vi "Stop.vi"(8 "error in (no error)":errorcluster, 10 "Message in":refnum<class "StopMessage.lvclass">, 11 "RSA in":refnum<class "RSA.lvclass">) -> (0 "error out":errorcluster, 3 "RSA out":refnum<class "RSA.lvclass">)   [LabVIEW 2012, in "RSA.lvclass"]
doc: "This member function is called when the statemachine in the run.vi receives an 'stop' command. It relays the message to all observers of the component.\n\nOverride this member function in your derived class if you need additional stop functionality (but don't forget to call the parent method)."
uses:
  RSA.lvclass
  <vilib>/Distrio/Murmex/StopMessage/StopMessage.lvclass
  <vilib>/Distrio/Murmex/Murmex/Murmex.lvclass
  RSA.lvclass/RSA.ctl
  <vilib>/Utility/file.llb/Write To Spreadsheet File (DBL).vi
panel:
  # "This method is called when the STOP\ntrigger is sent. \n\nOverride this method when your component needs to\nrespond to this trigger. \n\nCall parent for proper implementation"
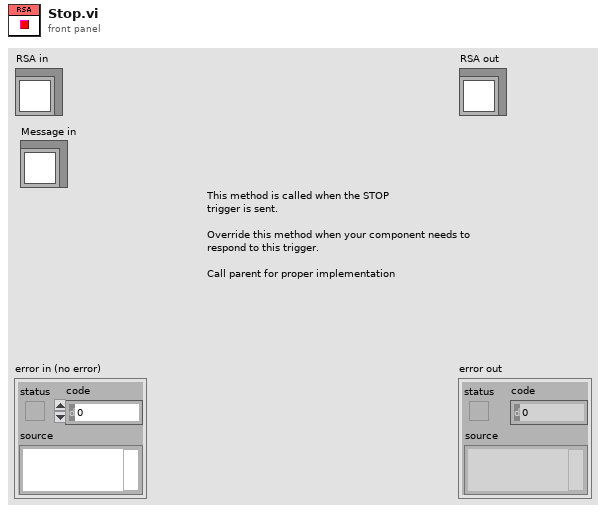
[diagram p1: front panel]
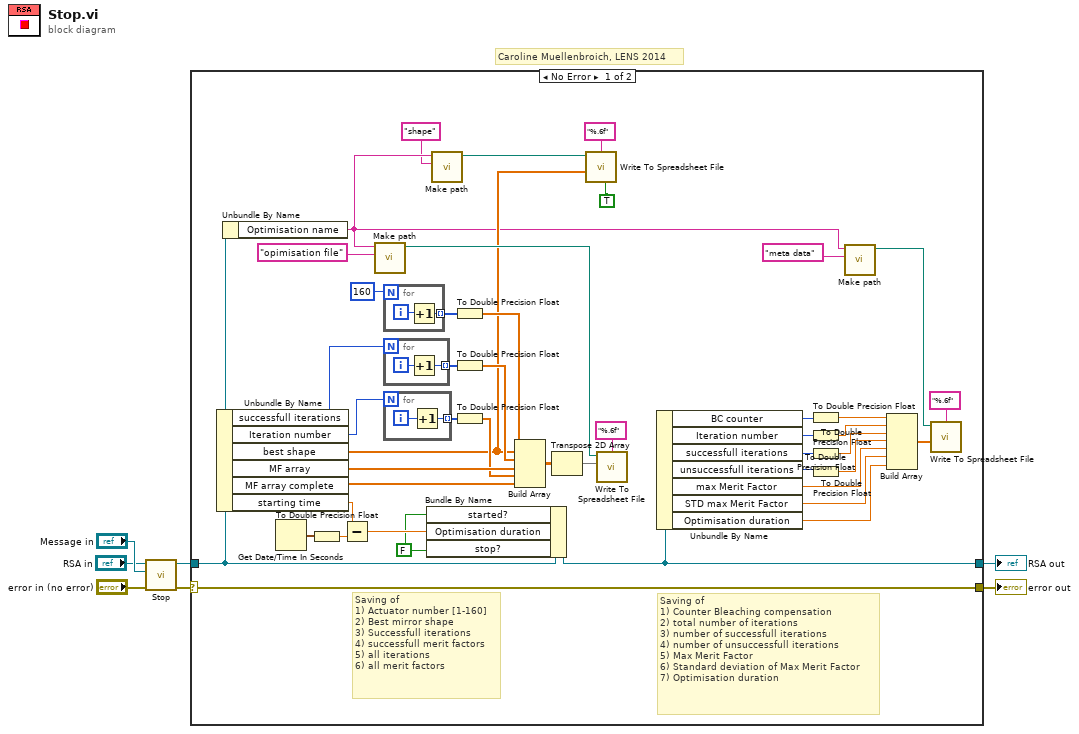
[diagram p0: block diagram]
diagram:
  # "Caroline Muellenbroich, LENS 2014"
  n1 = call-parent "Stop.vi"("error in (no error)"="error in (no error)", "Message in"="Message in", "Murmex in"="RSA in") -> ("error out"=w4:errorcluster, "Murmex out"=w2:refnum<class "RSA.lvclass">)  [unwired: 7 in]
  n2 = case shown="No Error" w4 {
    selector: w4 -> [w52 w59]
    tunnel: [w52 w59] -> w3
    tunnel: w2 -> [w34 w60]
    tunnel: [w31 w60] -> w1
    frame No Error {
      w8 = FALSE ("Run time cluster.stop?")
      # "Saving of\n1) Actuator number [1-160]\n2) Best mirror shape\n3) Successfull iterations\n4) successfull merit factors\n5) all iterations\n6) all merit factors"
      # "Saving of\n1) Counter Bleaching compensation\n2) total number of iterations\n3) number of successfull iterations\n4) number of unsuccessfull iterations\n5) Max Merit Factor\n6) Standard deviation of Max Merit Factor\n7) Optimisation duration"
      n3 = Unbundle By Name(w34) -> ("successfull iterations"=w43:i32, "Iteration number"=w40:i32, "best shape"=w12:dbl[], "MF array"=w38:dbl[], "MF array complete"=w36:dbl[], "starting time"=w50:dbl)
      n4 = Unbundle By Name(w34) -> ("Optimisation name"=w11:string)
      n5 = Get Date/Time In Seconds() -> (seconds since 1Jan1904=w51:timestamp)
      n6 = To Double Precision Float(number=w51) -> (double precision float=w49:dbl)
      n7 = Subtract(x=w50, y=w49) -> (x-y=w48:dbl)
      n8 = call "Make path.vi"("what?"="opimisation file" ("string"), "name"=w11) -> ("path"=w32:path)  [unwired: 9 in]
      n9 = for {
        N: 160 -> [_]
        tunnel: [w57] -> w46 mode=indexing
        i -> [w58]
        n10 = Increment(x=w58) -> (x+1=w57:i32)
      }
      n11 = for {
        N: w43 -> [_]
        tunnel: [w53] -> w42 mode=indexing
        i -> [w54]
        n12 = Increment(x=w54) -> (x+1=w53:i32)
      }
      n13 = for {
        N: w40 -> [_]
        tunnel: [w55] -> w44 mode=indexing
        i -> [w56]
        n14 = Increment(x=w56) -> (x+1=w55:i32)
      }
      n15 = Bundle By Name(cluster=w34, "started?"=w8, "Optimisation duration"=w48, "stop?"=w8) -> (w31:refnum<class "RSA.lvclass">)
      n16 = call "Make path.vi"("what?"="shape", "name"=w11) -> ("path"=w9:path)  [unwired: 9 in]
      n17 = To Double Precision Float(number=w46) -> (double precision float=w45:dbl[])
      n18 = To Double Precision Float(number=w42) -> (double precision float=w39:dbl[])
      n19 = To Double Precision Float(number=w44) -> (double precision float=w37:dbl[])
      n20 = Build Array(w45, w12, w39, w38, w37, w36) -> (w41:dbl[][])
      n21 = Transpose 2D Array(2D array=w41) -> (transposed array=w30:dbl[][])
      n22 = call-poly <vilib>:"Write To Spreadsheet File.vi"("transpose? (no:F)"=TRUE, "format (%.3f)"="%.6f", "1D data"=w12, "file path (dialog if empty)"=w9) -> ()  [unwired: 2 in, 3 out]
      n23 = call-poly <vilib>:"Write To Spreadsheet File.vi"("format (%.3f)"="%.6f", "2D data"=w30, "file path (dialog if empty)"=w32) -> ()  [unwired: 3 in, 3 out]
      n24 = Unbundle By Name(w31) -> ("BC counter"=w29:i32, "Iteration number"=w28:i32, "successfull iterations"=w27:i32, "unsuccessfull iterations"=w26:i32, "max Merit Factor"=w21:dbl, "STD max Merit Factor"=w20:dbl, "Optimisation duration"=w19:dbl)
      n25 = To Double Precision Float(number=w29) -> (double precision float=w25:dbl)
      n26 = To Double Precision Float(number=w28) -> (double precision float=w24:dbl)
      n27 = To Double Precision Float(number=w27) -> (double precision float=w23:dbl)
      n28 = To Double Precision Float(number=w26) -> (double precision float=w22:dbl)
      n29 = call "Make path.vi"("what?"="meta data" ("string"), "name"=w11) -> ("path"=w15:path)  [unwired: 9 in]
      n30 = Build Array(w25, w24, w23, w22, w21, w20, w19) -> (w17:dbl[])
      n31 = call-poly <vilib>:"Write To Spreadsheet File.vi"("format (%.3f)"="%.6f", "1D data"=w17, "file path (dialog if empty)"=w15) -> ()  [unwired: 3 in, 3 out]
    }
    frame Error {
    }
  }
  "error out" <- w3
  "RSA out" <- w1
